vi "getSelectedTasks.vi"(8 "error in (no error)":errorcluster, 10 "User Selections":string[](array[string]), 11 "BuildServer in":refnum<class "BuildServer.lvclass">) -> (0 "error out":errorcluster, 2 "Selected Tasks":refnum<class "Task.lvclass">[](array[class]), 3 "BuildServer out":refnum<class "BuildServer.lvclass">)   [LabVIEW 2017, in "BuildServer.lvlib" / "BuildServer.lvclass"]
uses:
  BuildServer.lvclass
  Classes/Task Interface/Task/Task.lvclass
  BuildServer.lvclass/BuildServer.ctl
  Classes/Task Interface/Task/Task.lvclass/Task.ctl
  Classes/Task Interface/Task/Get BuildSpec Name.vi
  <vilib>/BenjaminR/LookUp Table API/LUT.lvclass
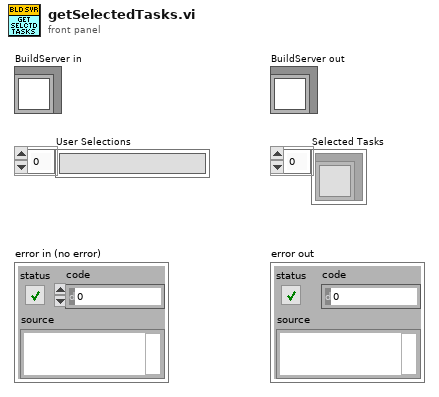
[diagram p1: front panel]
types:
  T1 = typedef "BuildServer.lvlib/BuildServer.lvclass/ProjectOrganization.ctl" = enum16{"Group by Project", "Group by Target", "Group by Type", "Group by Name"}
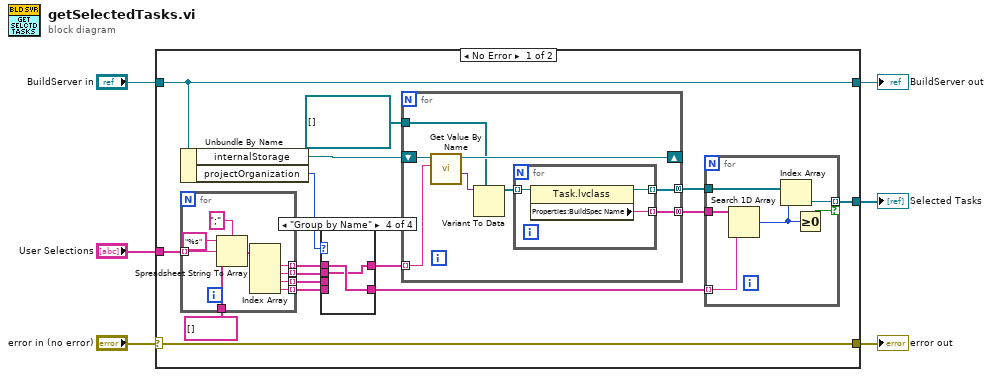
[diagram p0: block diagram]
diagram:
  n1 = case shown="No Error" "error in (no error)" {
    selector: "error in (no error)" -> [w22 w58]
    tunnel: [w22 w58] -> w2
    tunnel: [w21 w57] -> w4
    tunnel: "BuildServer in" -> [w21 w57]
    tunnel: "User Selections" -> [w19 _]
    tunnel: [w8 _] -> w6
    frame No Error {
      n2 = Unbundle By Name(w21) -> ("internalStorage"=w20:refnum<class "LUT.lvclass">, "projectOrganization"=w14:T1)
      n3 = for {
        tunnel: w19 -> [w49] mode=indexing
        tunnel: [w53] -> w18 mode=indexing
        tunnel: [w52] -> w17 mode=indexing
        tunnel: [w51] -> w16 mode=indexing
        tunnel: [w50] -> w15 mode=indexing
        tunnel: string[] [] -> [w56]
        n4 = Spreadsheet String To Array(delimiter (Tab)=";", format string="%s" ("spreadsheet string"), spreadsheet string=w49, array type (2D Dbl)=w56) -> (array=w54:string[])
        n5 = Index Array(array=w54) -> (element #1=w53:string, element #2=w52:string, element #3=w51:string, element #4=w50:string)  [unwired: 4 in]
      }
      n6 = case shown="\"Group by Name\"" w14 {
        tunnel: w18 -> [w41 _ _ w47]
        tunnel: w17 -> [_ w43 w44 w46]
        tunnel: w16 -> [_ _ _ _]
        tunnel: w15 -> [w40 w42 w45 _]
        tunnel: [w41 w43 w44 w46] -> w13
        tunnel: [w40 w42 w45 w47] -> w10
        frame "Group by Project", Default {
        }
        frame "Group by Target" {
        }
        frame "Group by Type" {
        }
        frame "Group by Name" {
        }
      }
      n7 = for {
        tunnel: w13 -> [w34] mode=indexing
        shift-right: [w35] -> _
        shift-left: w20 -> [w36]
        tunnel: refnum<class "Task.lvclass">[] [] -> [w32]
        tunnel: [w30] -> w11 mode=concatenating
        tunnel: [w29] -> w9 mode=concatenating
        n8 = call <vilib>:"Get Value By Name.vi"("Name"=w34, "LUT in"=w36) -> ("Value"=w33:variant, "LUT out"=w35:refnum<class "LUT.lvclass">)  [unwired: 6 in, 2 out]
        n9 = Variant To Data(type=w32, Variant=w33) -> (data=w31:refnum<class "Task.lvclass">[])  [unwired: 1 in, 1 out]
        n10 = for {
          tunnel: w31 -> [w39] mode=indexing
          tunnel: [w38] -> w30 mode=indexing
          tunnel: [w37] -> w29 mode=indexing
          n11 = property class="Task.lvclass"(reference=w39) -> (reference out=w37:refnum<class "Task.lvclass">, "Properties:BuildSpec Name"=w38:string)  [unwired: 1 in, 1 out]
        }
      }
      n12 = for {
        tunnel: w11 -> [w28]
        tunnel: w10 -> [w27] mode=indexing
        tunnel: w9 -> [w26]
        tunnel: [w25] -> w8 mode=indexing if=w23
        n13 = Search 1D Array(1D array=w28, element=w27) -> (index of element=w24:i32)  [unwired: 1 in]
        n14 = Index Array(array=w26, index=w24) -> (element=w25:refnum<class "Task.lvclass">)
        n15 = Greater Or Equal To 0?(x=w24) -> (x >= 0?=w23:bool)
      }
    }
    frame Error {
    }
  }
  "Selected Tasks" <- w6
  "BuildServer out" <- w4
  "error out" <- w2
